vi "20SimGenerateInputs.vi"(9 "InputArrayInitial":dbl[](array[numeric]), 10 "time in":dbl) -> (3 "InputArray":dbl[](array[numeric]))   [LabVIEW 2011]
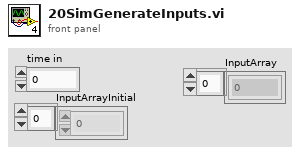
[diagram p1: front panel]
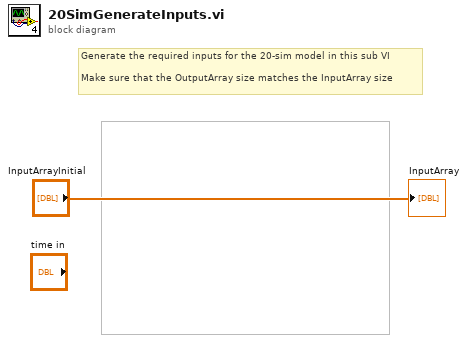
[diagram p0: block diagram]
diagram:
  # "Generate the required inputs for the 20-sim model in this sub VI\n\nMake sure that the OutputArray size matches the InputArray size"
  "InputArray" <- "InputArrayInitial"
